vi "Query Ethernet Autostart.vi"(0 "VISA resource name":refnum<visa-resource-name>, 11 "error in (no error)":errorcluster) -> (4 "VISA resource name out":refnum<visa-resource-name>, 6 "Autostart Enabled":bool, 15 "error out":errorcluster)   [LabVIEW 2020, in "eec EST 300.lvlib"]
doc: "Queries the Autostart Mode configured in the instrument"
uses:
  <instrlib>/eec EST 300/eec EST 300.lvlib
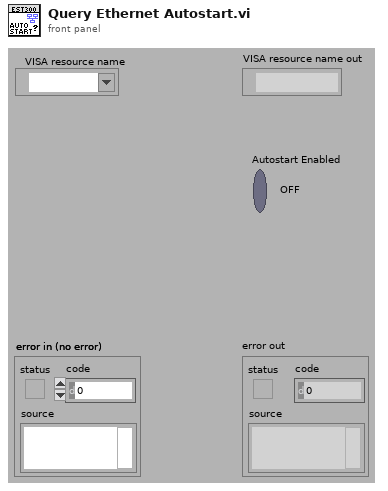
[diagram p1: front panel]
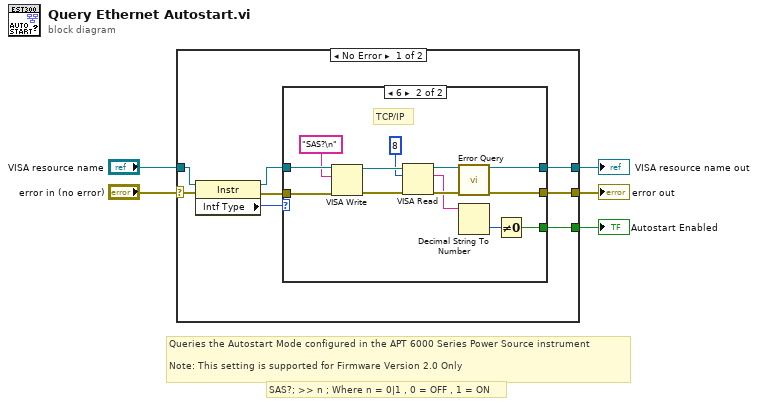
[diagram p0: block diagram]
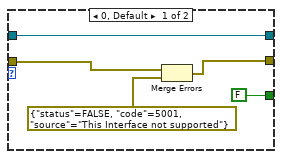
[diagram p2: hidden frame]
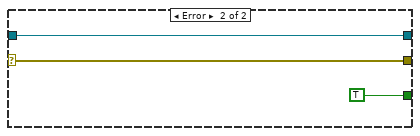
[diagram p3: hidden frame]
diagram:
  # "SAS?; >> n ; Where n = 0|1 , 0 = OFF , 1 = ON"
  # "Queries the Autostart Mode configured in the APT 6000 Series Power Source instrument\n\nNote: This setting is supported for Firmware Version 2.0 Only"
  n1 = case shown="No Error" "error in (no error)" {
    selector: "error in (no error)" -> [w11 w34]
    tunnel: [w13 w33] -> w4
    tunnel: [w12 w34] -> w5
    tunnel: "VISA resource name" -> [w7 w33]
    tunnel: [w6 TRUE ("Autostart Enabled")] -> w1
    frame No Error {
      n2 = property on="Property Node" class="Instr"(reference=w7, error in=w11) -> (reference out=w9:refnum<visa-resource-name>, error out=w10:errorcluster, "Intf Type"=w8:u16)
      n3 = case shown="6" w8 {
        tunnel: w9 -> [w18 w31]
        tunnel: [w18 w30] -> w13
        tunnel: [w17 w29] -> w12
        tunnel: w10 -> [w16 w27]
        tunnel: [FALSE w20] -> w6
        frame 0, Default {
          n4 = Merge Errors(w16, errorcluster {"status"=FALSE, "code"=5001, "source"="This Interface not supported"} ("error in 2 (no error)")) -> (w17:errorcluster)
        }
        frame 6 {
          # "TCP/IP"
          n5 = VISA Write(VISA resource name=w31, write buffer="SAS?\n" ("Command to Send"), error in (no error)=w27) -> (VISA resource name out=w25:refnum<visa-resource-name>, error out=w26:errorcluster)  [unwired: 1 out]
          n6 = VISA Read(VISA resource name=w25, byte count=u32 8, error in (no error)=w26) -> (VISA resource name out=w24:refnum<visa-resource-name>, read buffer=w19:string, error out=w23:errorcluster)  [unwired: 1 out]
          n7 = call <instrlib>:"Error Query.vi"("VISA resource name"=w24, "error in (no error)"=w23) -> ("VISA resource name out"=w30:refnum<visa-resource-name>, "error out"=w29:errorcluster)  [unwired: 10 in, 2 out]
          n8 = Decimal String To Number(string=w19) -> (number=w22:i32)  [unwired: 2 in, 1 out]
          n9 = Not Equal To 0?(x=w22) -> (x != 0?=w20:bool)
        }
      }
    }
    frame Error {
    }
  }
  "error out" <- w5
  "VISA resource name out" <- w4
  "Autostart Enabled" <- w1
